vi "Progress Bar - UI.vi"(8 "error in (no error)":errorcluster, 9 "Number of Steps":dbl, 11 "Ref Cluster":T1) -> (0 "error out":errorcluster)   [LabVIEW 2014, in "Progress Bar.lvlib"]
uses:
  Progress Bar.lvlib
  _typedefs/PB_Ref Cluster.ctl
panel:
  in  "Cancel":bool
  out "Message History":string
  out "Progress Bar":u8(slide) scale=0.0..5.0
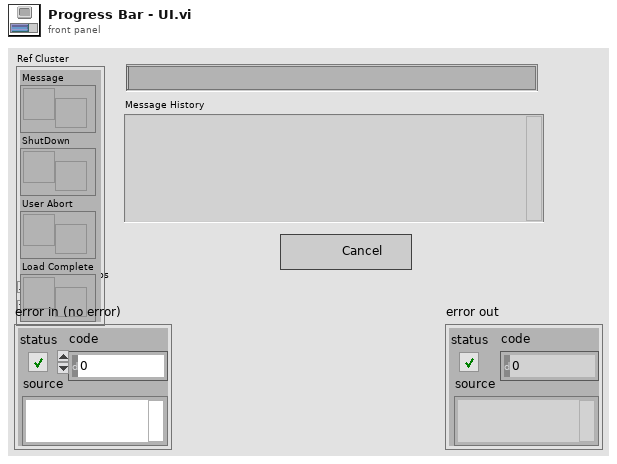
[diagram p1: front panel]
types:
  T1 = typedef "PB_Ref Cluster.ctl" = cluster{"Message":refnum<user-event>, "ShutDown":refnum<user-event>, "User Abort":refnum<notifier>, "Load Complete":refnum<notifier>}
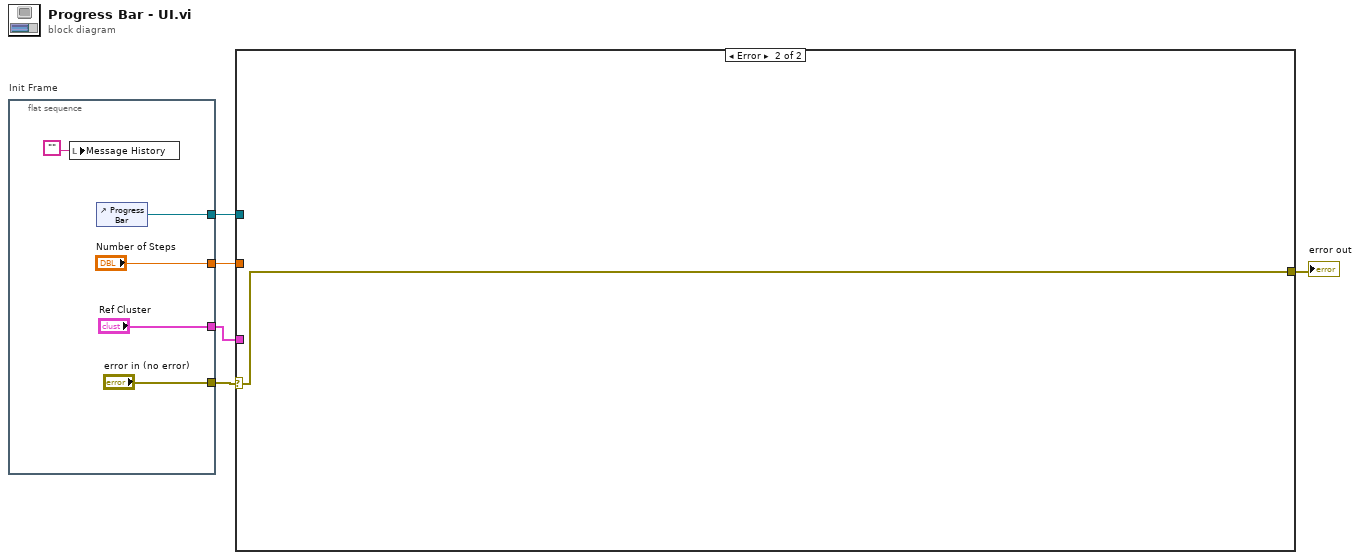
[diagram p0: block diagram]
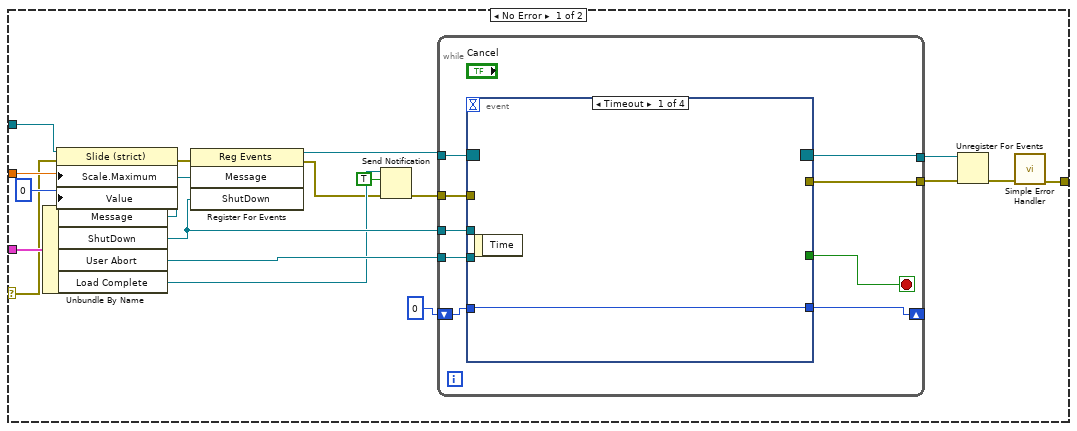
[diagram p2: hidden frame]
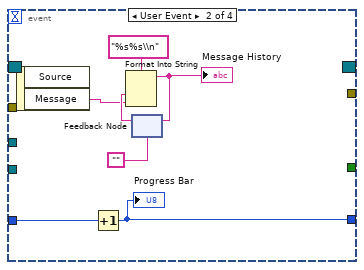
[diagram p3: hidden frame]
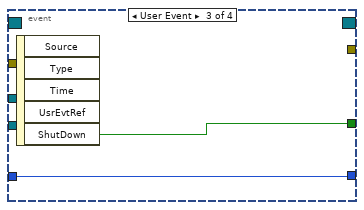
[diagram p4: hidden frame]
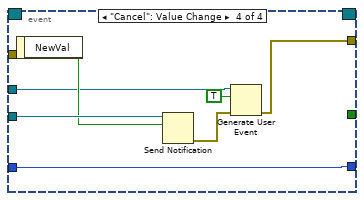
[diagram p5: hidden frame]
diagram:
  n1 = flat-sequence "Init Frame" {
    tunnel: ["Number of Steps"] -> w5
    tunnel: ["Ref Cluster"] -> w4
    tunnel: [w7] -> w3
    tunnel: ["error in (no error)"] -> w1
    frame #0 {
      n2 = local write "Message History"("") -> ()
      n3 = control-ref of="Progress Bar"() -> (w7:refnum<vi>)
    }
  }
  n4 = case shown="Error" w1 {
    selector: w1 -> [w11 w56]
    tunnel: w5 -> [w29 _]
    tunnel: w4 -> [w26 _]
    tunnel: w3 -> [w18 _]
    tunnel: [w14 w56] -> w2
    frame No Error {
      n5 = Unbundle By Name(w26) -> ("Message"=w25:refnum<user-event>, "ShutDown"=w23:refnum<user-event>, "User Abort"=w24:refnum<notifier>, "Load Complete"=w17:refnum<notifier>)
      n6 = property class="Slide (strict)"(reference=w18, error in=w11, "Scale.Maximum"=w29, "Value"=u8 0) -> (error out=w27:errorcluster)  [unwired: 1 out]
      n7 = register-events(error in=w27, w25, w23) -> (reference out=w28:refnum<event-registration>, error out=w16:errorcluster)  [unwired: 1 in]
      n8 = Send Notification(notification=TRUE, notifier=w17, error in (no error)=w16) -> (error out=w15:errorcluster)  [unwired: 1 out]
      n9 = while {
        tunnel: w28 -> [w38]
        tunnel: w24 -> [w36]
        tunnel: w23 -> [w35]
        tunnel: [w34] -> w22
        tunnel: [w33] -> w20
        shift-right: [w31] -> _
        shift-left: u8 0 -> [w32]
        tunnel: w15 -> [w30]
        stop <- w37 stop-if-true
        n10 = event shown="[0] Timeout" {
          selector: w38 -> [_ _ _ _]
          dyn-events: [_ _ _ _] -> w34
          timeout: _ -> [_ _ _ _]
          tunnel: [_ _ w48 _] -> w37
          tunnel: w36 -> [_ _ _ w55]
          tunnel: w35 -> [_ _ _ w52]
          tunnel: [_ _ _ w50] -> w33
          tunnel: w32 -> [w39 w41 w47 w49]
          tunnel: [w39 w40 w47 w49] -> w31
          tunnel: w30 -> [_ _ _ _]
          event Timeout {
            n11 = event-data() -> ()  [unwired: 1 in, 1 out]
          }
          event User Event {
            n12 = event-data() -> ("Message"=w44:string)  [unwired: 1 in, 1 out]
            n13 = Increment(x=w41) -> (x+1=w40:u8)
            "Progress Bar" <- w40
            n14 = feedback #1("") -> (w45:string)
            n15 = Format Into String(format string="%s%s\\n", w45, w44) -> (resulting string=w43:string)  [unwired: 2 in, 1 out]
            "Message History" <- w43
            n16 = feedback-in #1(w43) -> ()
          }
          event User Event {
            n17 = event-data() -> ("ShutDown"=w48:bool)  [unwired: 1 in, 4 out]
          }
          event "Cancel": Value Change {
            n18 = event-data() -> ("NewVal"=w54:bool)  [unwired: 1 in]
            n19 = Send Notification(notification=w54, notifier=w55) -> (error out=w53:errorcluster)  [unwired: 1 in, 1 out]
            n20 = Generate User Event(user event=w52, event data cluster=TRUE ("event data"), error in=w53) -> (error out=w50:errorcluster)  [unwired: 1 in, 1 out]
          }
        }
      }
      n21 = Unregister For Events(event registration refnum=w22, error in=w20) -> (error out=w21:errorcluster)
      n22 = call <vilib>:"Simple Error Handler.vi"("error in (no error)"=w21) -> ("error out"=w14:errorcluster)  [unwired: 4 in, 4 out]
    }
    frame Error {
    }
  }
  "error out" <- w2
